vi "Controller Test Bench (7).vi"() -> ()   [LabVIEW 2022 SP3]
uses:
  WhiteNoise.ctl
  <vilib>/sound2/lvsound2.llb/Sound Data Format.ctl
  <vilib>/Utility/error.llb/DialogType.ctl
  <vilib>/sound2/lvsound2.llb/Sampling Mode.ctl
  <vilib>/Analysis/4window.llb/windowTd.ctl
  <vilib>/DAQmx/write.llb/DAQmx Write (Analog 1D Wfm NChan NSamp).vi
  <vilib>/DAQmx/read.llb/DAQmx Read (Analog 1D Wfm NChan NSamp).vi
  <vilib>/DAQmx/create/channels.llb/DAQmx Create Channel (AO-Voltage-Basic).vi
  <vilib>/DAQmx/create/channels.llb/DAQmx Create Channel (AI-Acceleration-Accelerometer).vi
  <vilib>/DAQmx/configure/timing.llb/DAQmx Timing (Sample Clock).vi
  <vilib>/DAQmx/miscellaneous.llb/DAQmx Fill In Error Info.vi
  <vilib>/sound2/lvsound2.llb/Sound Output Set Volume (Single).vi
  <vilib>/sound2/lvsound2.llb/Sound Output Write (DBL).vi
  <vilib>/DAQmx/configure/task.llb/DAQmx Configure Logging (TDMS).vi
  <vilib>/measure/maspectr.llb/FFT Spectrum (Mag-Phase) for N Chan.vi
  <vilib>/measure/NI_MAPro.lvlib
  <resource>/objmgr/daqmx.rc
  <vilib>/Analysis/NI_AALPro.lvlib
  <vilib>/measure/NI_MABase.lvlib
panel:
  in  "?":enum32{"White Noise", "Harmonic"}(tab)
  in  "Cluster":T2={"Seed"=0.0, "Standard Deviation"=0.2, "Reset"=FALSE, "Iterator"=1.0} {"Standard Deviation" format="%0.2p"}
  in  "Cluster 2":T3={"Iterator"=1.0, "Waveform Type"=0, "Frequency"=10.0, "Amplitude"=0.5} {"Frequency" format="%0.2p"; "Waveform Type" items=["Sine Wave", "Triangle Wave", "Square Wave", "Sawtooth Wave"]; "Amplitude" format="%0.2p"}
  in  "Number of Samples":i32=41200
  out "Actual Sample Rate":dbl=1000.0 format="%0.2f"
  in  "Output Noise":bool
  out "Accel.1":waveform(dbl)[](graph)
  out "Accel.2":waveform(dbl)[](graph)
  in  "Setpoint":dbl
  in  "Gain":dbl min=0.0 step=0.01
  in  "Active Control":bool
  in  "Log Data":bool
  out "Phase 2":cluster{"f0":dbl, "df":dbl, "phase":dbl[]}[](graph)
  out "Mag 2":cluster{"f0":dbl, "df":dbl, "magnitude":dbl[]}[](graph)
  in  "Show FFT":bool
  in  "Save FFT":bool
  in  "Start Acquisition":bool
  in  "Stop":bool
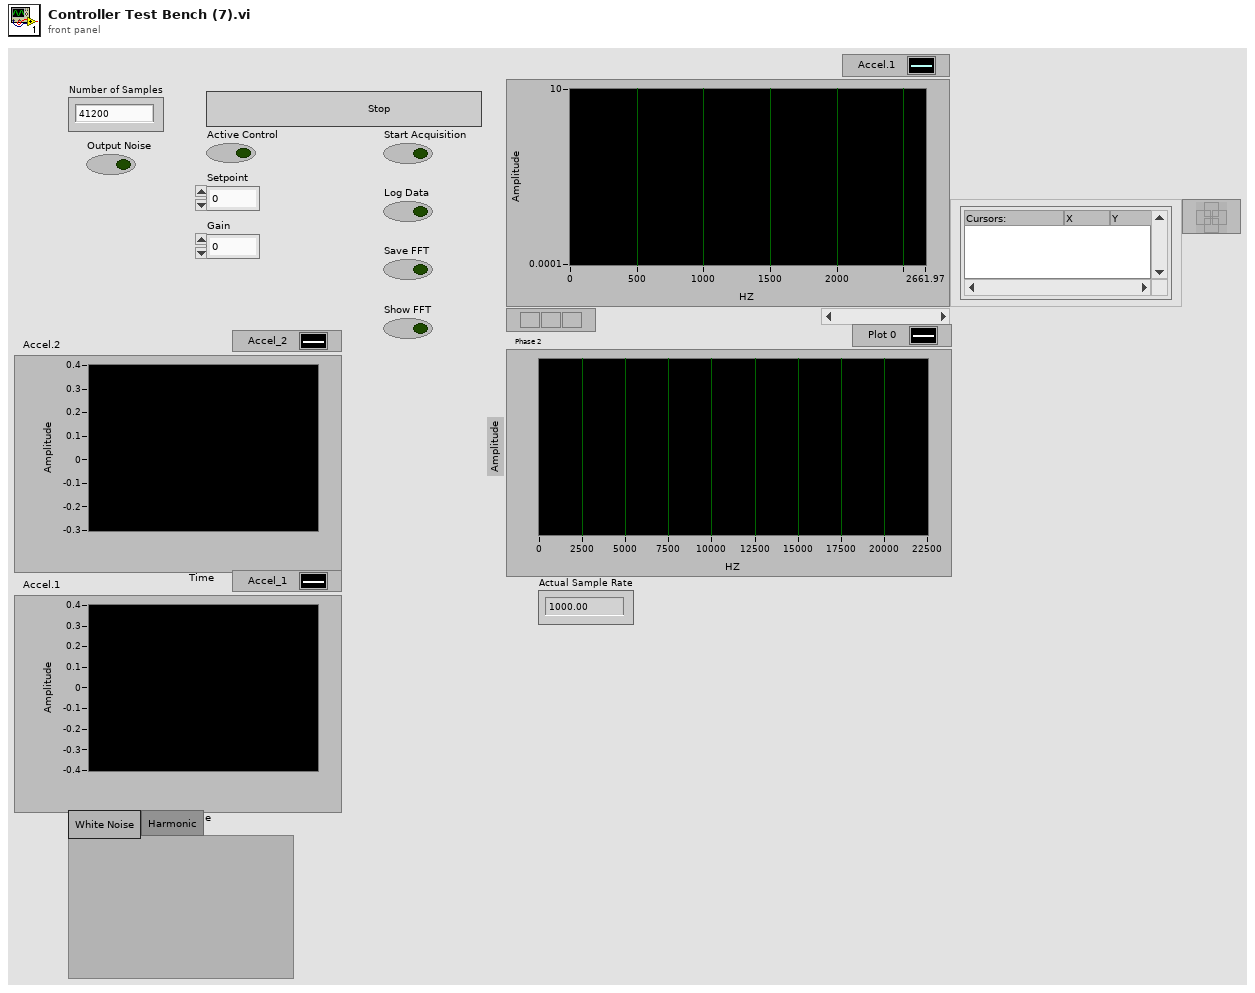
[diagram p1: front panel]
types:
  T1 = typedef "WhiteNoise.ctl" = dbl
  T2 = cluster{"Seed":T1, "Standard Deviation":dbl, "Reset":bool, "Iterator":dbl}
  T3 = cluster{"Iterator":dbl, "Waveform Type":u16, "Frequency":dbl, "Amplitude":dbl}
  T4 = typedef "Sampling Mode.ctl" = i32
  T5 = typedef "DialogType.ctl" = u16
  T6 = typedef "Sound Data Format.ctl" = cluster{"sample rate (S/s)":dbl, "number of channels":i32, "bits per sample":i32}
  T7 = typedef "Sound Output Task ID.ctl" = u32
  T8 = typedef "NI_AALPro.lvlib/windowTd.ctl" = u32
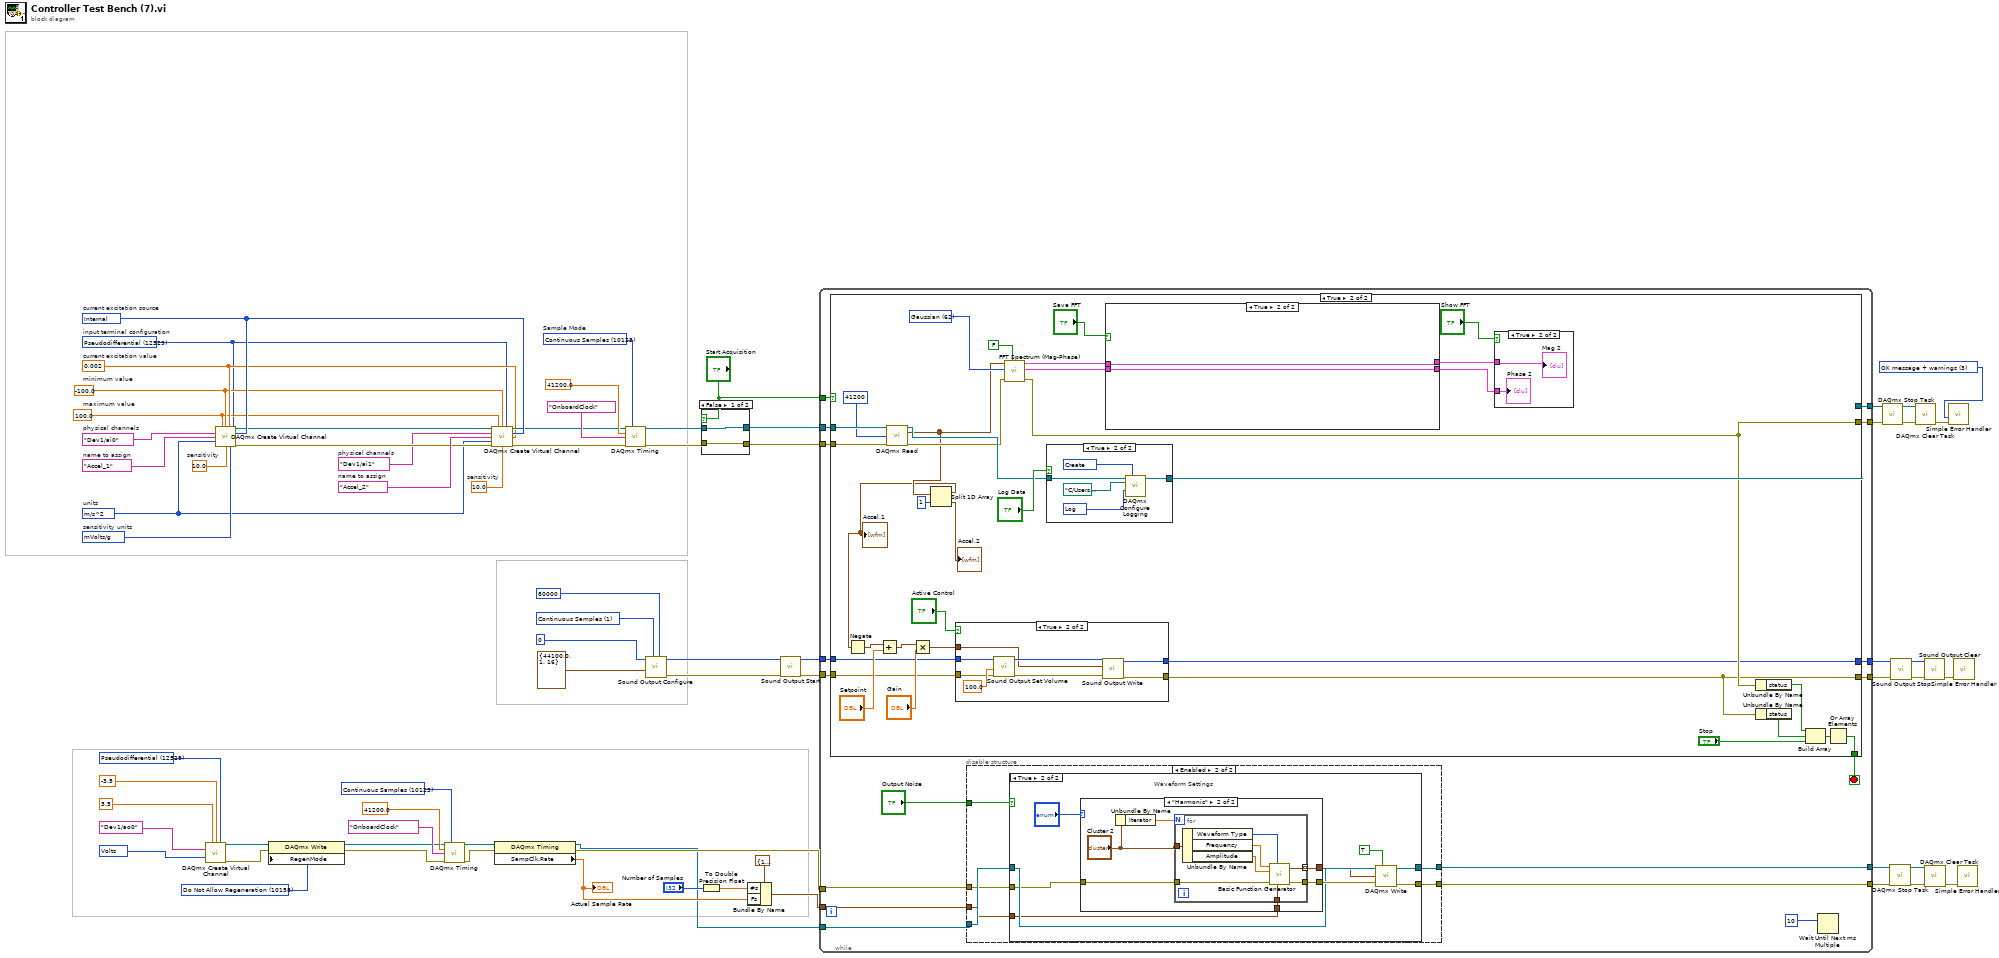
[diagram p0: block diagram]
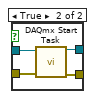
[diagram p2: hidden frame]
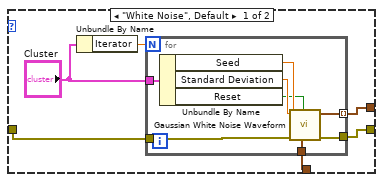
[diagram p5: hidden frame]
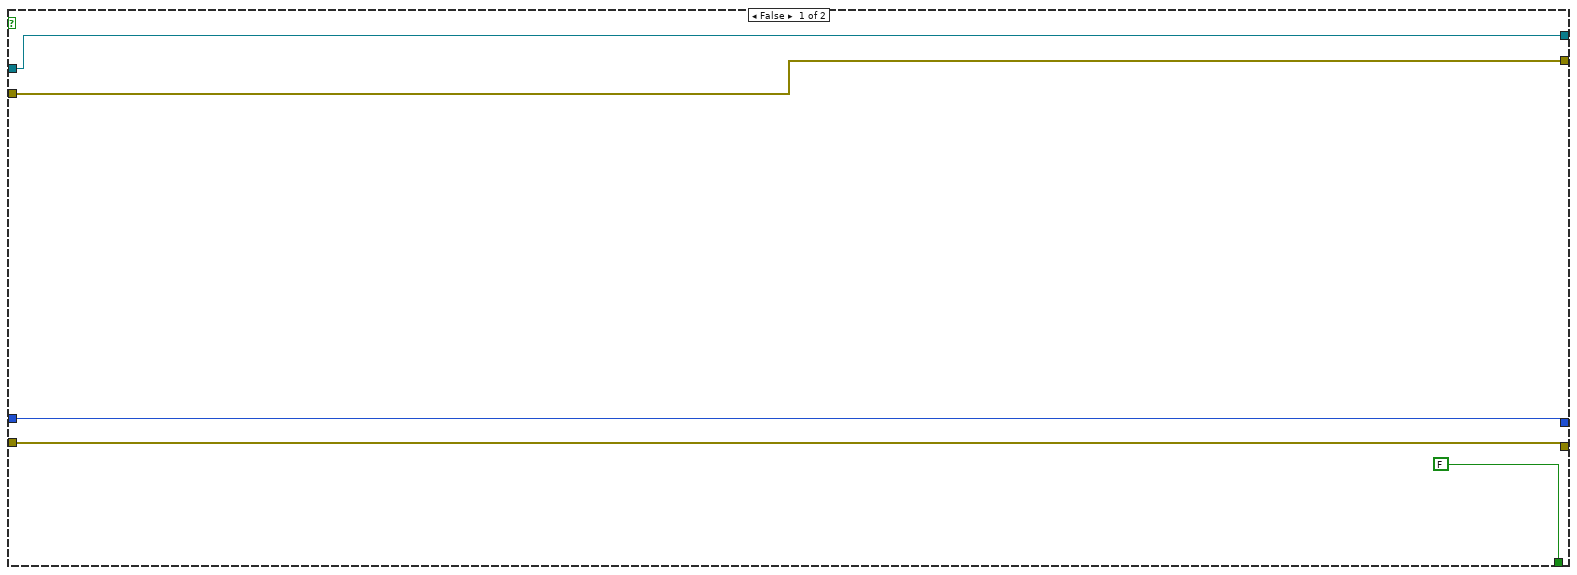
[diagram p6: hidden frame]
diagram:
  w39 = 10123 items=["Finite Samples"=10178, "Continuous Samples"=10123, "Hardware Timed Single Point"=12522] ("sample mode")
  w43 = 12509 items=["mVolts/g"=12509, "Volts/g"=12510]  # sensitivity units
  w44 = 10.0  # sensitivity
  w33 = 0.002  # current excitation value
  w36 = 10200 items=["Internal"=10200, "External"=10167, "None"=10230]  # current excitation source
  w26 = tag "Dev1/ai0"  # physical channels
  w42 = 10123 items=["Finite Samples"=10178, "Continuous Samples"=10123, "Hardware Timed Single Point"=12522]  # Sample Mode
  w29 = 12529 items=["default"=-1, "RSE"=10083, "NRSE"=10078, "Differential"=10106, "Pseudodifferential"=12529]  # input terminal configuration
  w32 = -100.0  # minimum value
  w31 = 100.0  # maximum value
  w45 = "Accel_1"  # name to assign
  w30 = 12470 items=["g"=10186, "m/s^2"=12470, "in/s^2"=12471, "From Custom Scale"=10065]  # units
  w46 = 10.0  # sensitivity
  w27 = tag "Dev1/ai1"  # physical channels
  w38 = "Accel_2"  # name to assign
  w47 = T4 1 items=["Finite Samples", "Continuous Samples"] ("sample mode")
  w53 = 10158 items=["Allow Regeneration"=10097, "Do Not Allow Regeneration"=10158] ("RegenMode")
  w48 = T5 3 items=["no dialog", "OK message", "continue or stop message", "OK message + warnings", "continue/stop + warnings"] ("type of dialog (OK msg:1)")
  w66 = 12529 items=["Default"=-1, "RSE"=10083, "Differential"=10106, "Pseudodifferential"=12529] ("output terminal configuration")
  w64 = 10348 items=["Volts"=10348, "From Custom Scale"=10065] ("units")
  n1 = call-poly <vilib>:"DAQmx Create Virtual Channel.vi"("maximum value"=3.5, "minimum value"=-3.5, "output terminal configuration"=w66, "physical channels"=tag "Dev1/ao0", "units"=w64) -> ("task out"=w52:refnum<k21>, "error out"=w54:errorcluster)  [unwired: 9 in]
  n2 = call-poly <vilib>:"DAQmx Create Virtual Channel.vi"("maximum value"=w31, "minimum value"=w32, "input terminal configuration"=w29, "physical channels"=w26, "current excitation source"=w36, "name to assign"=w45, "current excitation value"=w33, "units"=w30, "sensitivity"=w44, "sensitivity units"=w43) -> ("task out"=w28:refnum<k21>, "error out"=w37:errorcluster)  [unwired: 4 in]
  n3 = property class="DAQmx Write"(reference=w52, error in=w54, "RegenMode"=w53) -> (reference out=w50:refnum<k21>, error out=w51:errorcluster)
  n4 = call-poly <vilib>:"DAQmx Timing.vi"("task/channels in"=w50, "sample mode"=w39, "rate"=41200.0 ("Sample Rate"), "source"=tag "OnboardClock" ("Sample Clock Source"), "error in"=w51) -> ("task out"=w10:refnum<k21>, "error out"=w9:errorcluster)  [unwired: 9 in]
  n5 = call-poly <vilib>:"DAQmx Create Virtual Channel.vi"("task in"=w28, "maximum value"=w31, "minimum value"=w32, "input terminal configuration"=w29, "physical channels"=w27, "current excitation source"=w36, "name to assign"=w38, "current excitation value"=w33, "units"=w30, "error in"=w37, "sensitivity"=w46) -> ("task out"=w35:refnum<k21>, "error out"=w34:errorcluster)  [unwired: 3 in]
  n6 = property class="DAQmx Timing"(reference=w10, error in=w9) -> (reference out=w6:refnum<k21>, error out=w8:errorcluster, "SampClk.Rate"=w11:dbl)
  "Actual Sample Rate" <- w11
  n7 = call-poly <vilib>:"DAQmx Timing.vi"("task/channels in"=w35, "sample mode"=w42, "rate"=41200.0 ("Sample Rate"), "source"=tag "OnboardClock" ("Sample Clock Source"), "error in"=w34) -> ("task out"=w24:refnum<k21>, "error out"=w25:errorcluster)  [unwired: 9 in]
  n8 = call <vilib>:"Sound Output Configure.vi"("number of samples/ch"=80000 ("Number of Samples/ch"), "sample mode"=w47, "sound format"=T6 {"sample rate (S/s)"=44100.0, "number of channels"=1, "bits per sample"=16} ("Sound Format"), "device ID"=u32 0 ("Device ID")) -> ("error out"=w18:errorcluster, "task ID"=w17:T7)  [unwired: 6 in]
  n9 = To Double Precision Float(number="Number of Samples") -> (double precision float=w13:dbl)
  n10 = case shown="False" "Start Acquisition" {
    tunnel: w25 -> [w72 w77]
    tunnel: w24 -> [w73 w76]
    tunnel: [w73 w75] -> w63
    tunnel: [w72 w74] -> w62
    frame False {
    }
    frame True {
      n11 = call <vilib>:"DAQmx Start Task.vi"("task/channels in"=w76, "error in"=w77) -> ("task out"=w75:refnum<k21>, "error out"=w74:errorcluster)  [unwired: 12 in]
    }
  }
  n12 = Bundle By Name(cluster=cluster{"Fs":dbl, "#s":dbl} {"Fs"=1000.0, "#s"=1000.0} ("sampling info"), "#s"=w13, "Fs"=w11) -> (w7:cluster{"Fs":dbl, "#s":dbl})
  n13 = call <vilib>:"Sound Output Start.vi"("error in (no error)"=w18, "task ID"=w17) -> ("error out"=w15:errorcluster, "task ID out"=w16:T7)  [unwired: 8 in]
  n14 = while {
    tunnel: w63 -> [w93]
    tunnel: w62 -> [w92]
    tunnel: [w90] -> w58
    tunnel: [w91] -> w57
    tunnel: "Start Acquisition" -> [w89]
    tunnel: [w84] -> w20
    tunnel: [w85] -> w19
    tunnel: w16 -> [w87]
    tunnel: w15 -> [w86]
    tunnel: w8 -> [w82]
    tunnel: w7 -> [w81]
    tunnel: w6 -> [w80]
    tunnel: [w79] -> w3
    tunnel: [w78] -> w2
    stop <- w94 stop-if-true
    n15 = case shown="True" w89 {
      tunnel: [FALSE w179] -> w94
      tunnel: w93 -> [w144 w178]
      tunnel: w92 -> [w143 w177]
      tunnel: [w144 w174] -> w91
      tunnel: [w143 w162] -> w90
      tunnel: w87 -> [w140 w148]
      tunnel: w86 -> [w141 w147]
      tunnel: [w140 w146] -> w85
      tunnel: [w141 w145] -> w84
      frame False {
      }
      frame True {
        w161 = T8 62 items=["Rectangle"=0, "Hanning"=1, "Hamming"=2, "Blackman-Harris"=3, "Exact Blackman"=4, "Blackman"=5, "Flat Top"=6, "4 Term B-Harris "=7, "7 Term B-Harris"=8, "Low Sidelobe"=9, "Blackman Nuttall"=11, "Triangle"=30, "Bartlett-Hanning"=31, "Bohman"=32, "Parzen"=33, "Welch"=34, "Kaiser"=60, "Dolph-Chebyshev"=61, "Gaussian"=62] ("window")
        n16 = call-poly <vilib>:"DAQmx Read.vi"("task/channels in"=w178, "number of samples per channel"=41200, "error in"=w177) -> ("task out"=w175:refnum<k21>, "data"=w154:waveform(dbl)[], "error out"=w163:errorcluster)  [unwired: 10 in]
        n17 = Split 1D Array(array=w154, index=1) -> (first subarray=w149:waveform(dbl)[], second subarray=→"Accel.2":waveform(dbl)[])
        "Accel.1" <- w149
        n18 = Negate(x=w149) -> (-x=w156:waveform(dbl)[])
        n19 = Add(x=w156, y="Setpoint") -> (x+y=w157:waveform(dbl)[])
        n20 = Multiply(x=w157, y="Gain") -> (x*y=w150:waveform(dbl)[])
        n21 = case shown="True" "Active Control" {
          tunnel: w147 -> [w181 w187]
          tunnel: [w181 w183] -> w145
          tunnel: w150 -> [_ w184]
          tunnel: w148 -> [w180 w188]
          tunnel: [w180 w182] -> w146
          frame False {
          }
          frame True {
            n22 = call-poly <vilib>:"Sound Output Set Volume.vi"("error in (no error)"=w187, "volume"=100.0, "task ID"=w188) -> ("error out"=w185:errorcluster, "task ID out"=w186:T7)  [unwired: 7 in]
            n23 = call-poly <vilib>:"Sound Output Write.vi"("error in (no error)"=w185, "data"=w184, "task ID"=w186) -> ("error out"=w183:errorcluster, "task ID out"=w182:T7)  [unwired: 7 in]
          }
        }
        n24 = call-poly <vilib>:"FFT Spectrum (Mag-Phase).vi"("restart averaging (F)"=FALSE, "error in (no error)"=w163, "window"=w161, "time signals"=w154) -> ("error out"=w162:errorcluster, "phases"=w168:cluster{"f0":dbl, "df":dbl, "phase":dbl[]}[], "magnitudes"=w169:cluster{"f0":dbl, "df":dbl, "magnitude":dbl[]}[])  [unwired: 3 in, 2 out]
        n25 = case shown="True" "Log Data" {
          tunnel: w175 -> [w196 w198]
          tunnel: [w196 w197] -> w174
          frame False {
          }
          frame True {
            w199 = 15848 items=["Open"=10437, "Open or Create"=15846, "Create or Replace"=15847, "Create"=15848] ("operation")
            w200 = 15844 items=["Off"=10231, "Log"=15844, "Log and Read"=15842] ("logging mode")
            n26 = call-poly <vilib>:"DAQmx Configure Logging.vi"("task/channels in"=w198, "operation"=w199, "file path"=path "C:/Users/LAV-UFSC/Documents/LAV - TCC", "logging mode"=w200) -> ("task out"=w197:refnum<k21>)  [unwired: 10 in, 1 out]
          }
        }
        n27 = case shown="True" "Save FFT" {
          tunnel: w169 -> [w190 w193]
          tunnel: w168 -> [w191 w192]
          tunnel: [w191 w192] -> w167
          tunnel: [w190 w193] -> w166
          frame False {
          }
          frame True {
          }
        }
        n28 = case shown="True" "Show FFT" {
          tunnel: w166 -> [_ w195]
          tunnel: w167 -> [_ w194]
          frame False {
          }
          frame True {
            "Mag 2" <- w195
            "Phase 2" <- w194
          }
        }
        n29 = Unbundle By Name(w162) -> ("status"=w159:bool)
        n30 = Unbundle By Name(w145) -> ("status"=w165:bool)
        n31 = Build Array(w159, w165, "Stop") -> (w172:bool[])
        n32 = Or Array Elements(Boolean array=w172) -> (logical OR=w179:bool)
      }
    }
    n33 = disable-structure shown="Enabled" {
      disable-tunnel: "Output Noise" -> [_ w96]
      disable-tunnel: w82 -> [_ w97]
      disable-tunnel: w81 -> [_ w95]
      disable-tunnel: w80 -> [_ w98]
      disable-tunnel: [_ w99] -> w79
      disable-tunnel: [_ w100] -> w78
      frame Disabled {
      }
      frame Enabled {
        n34 = case shown="True" w96 {
          tunnel: [w102 w109] -> w100
          tunnel: [w101 w108] -> w99
          tunnel: w98 -> [w102 w107]
          tunnel: w97 -> [w101 w105]
          tunnel: w95 -> [_ w106]
          frame False {
          }
          frame True {
            # "Waveform Settings"
            n35 = case shown="\"Harmonic\"" "?" {
              tunnel: w106 -> [w117 w129]
              tunnel: w105 -> [w112 w131]
              tunnel: [w116 w128] -> w110
              tunnel: [w113 w130] -> w104
              frame "White Noise", Default {
                n36 = Unbundle By Name("Cluster") -> ("Iterator"=w115:dbl)
                n37 = for {
                  N: w115 -> [_]
                  tunnel: w112 -> [w125]
                  tunnel: w117 -> [w124]
                  tunnel: [w123] -> w116
                  tunnel: "Cluster" -> [w122]
                  tunnel: [w121] -> w113 mode=indexing
                  n38 = Unbundle By Name(w122) -> ("Seed"=w120:T1, "Standard Deviation"=w119:dbl, "Reset"=w118:bool)
                  n39 = call <vilib>:"Gaussian White Noise Waveform.vi"("sampling info"=w124, "reset signal"=w118, "error in (no error)"=w125, "seed"=w120, "standard deviation"=w119) -> ("error out"=w123:errorcluster, "signal out"=w121:waveform(dbl))  [unwired: 5 in]
                }
              }
              frame "Harmonic" {
                n40 = Unbundle By Name("Cluster 2") -> ("Iterator"=w127:dbl)
                n41 = for {
                  N: w127 -> [_]
                  tunnel: w131 -> [w139]
                  tunnel: w129 -> [w138]
                  tunnel: [w137] -> w128
                  tunnel: "Cluster 2" -> [w136]
                  tunnel: [w132] -> w130 mode=indexing
                  n42 = Unbundle By Name(w136) -> ("Waveform Type"=w135:u16, "Frequency"=w134:dbl, "Amplitude"=w133:dbl)
                  n43 = call <vilib>:"Basic Function Generator.vi"("sampling info"=w138, "signal type"=w135, "error in (no error)"=w139, "amplitude"=w133, "frequency"=w134) -> ("error out"=w137:errorcluster, "signal out"=w132:waveform(dbl))  [unwired: 4 in, 1 out]
                }
              }
            }
            n44 = call-poly <vilib>:"DAQmx Write.vi"("task/channels in"=w107, "auto start"=TRUE, "data"=w104, "error in"=w110) -> ("task out"=w109:refnum<k21>, "error out"=w108:errorcluster)  [unwired: 9 in, 1 out]
          }
        }
      }
    }
    n45 = Wait Until Next ms Multiple(millisecond multiple=u32 10) -> ()  [unwired: 1 out]
  }
  n46 = call <vilib>:"DAQmx Stop Task.vi"("task/channels in"=w57, "error in"=w58) -> ("task out"=w60:refnum<k21>, "error out"=w59:errorcluster)  [unwired: 12 in]
  n47 = call <vilib>:"DAQmx Stop Task.vi"("task/channels in"=w2, "error in"=w3) -> ("task out"=w5:refnum<k21>, "error out"=w4:errorcluster)  [unwired: 12 in]
  n48 = call <vilib>:"Sound Output Stop.vi"("error in (no error)"=w20, "task ID"=w19) -> ("error out"=w23:errorcluster, "task ID out"=w22:T7)  [unwired: 8 in]
  n49 = call <vilib>:"DAQmx Clear Task.vi"("task in"=w60, "error in"=w59) -> ("error out"=w61:errorcluster)  [unwired: 13 in]
  n50 = call <vilib>:"Sound Output Clear.vi"("error in (no error)"=w23, "task ID"=w22) -> ("error out"=w21:errorcluster)  [unwired: 9 in]
  n51 = call <vilib>:"DAQmx Clear Task.vi"("task in"=w5, "error in"=w4) -> ("error out"=w1:errorcluster)  [unwired: 13 in]
  n52 = call <vilib>:"Simple Error Handler.vi"("type of dialog (OK msg:1)"=w48, "error in (no error)"=w61) -> ()  [unwired: 3 in, 5 out]
  n53 = call <vilib>:"Simple Error Handler.vi"("error in (no error)"=w21) -> ()  [unwired: 4 in, 5 out]
  n54 = call <vilib>:"Simple Error Handler.vi"("error in (no error)"=w1) -> ()  [unwired: 4 in, 5 out]
